vi "string_to_numberVariant.vi"(11 "String":string) -> (0 "error out":errorcluster, 3 "Variant":variant)   [LabVIEW 2014]
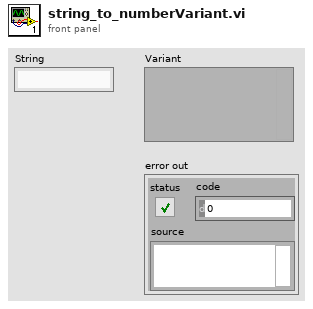
[diagram p1: front panel]
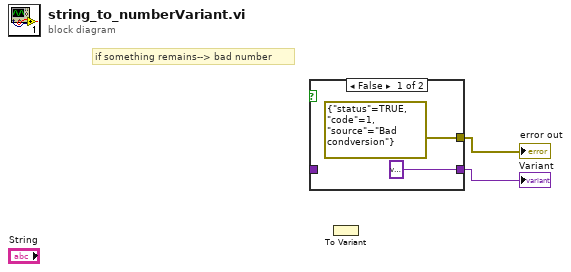
[diagram p0: block diagram]
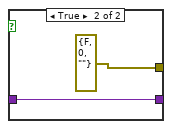
[diagram p2: hidden frame]
diagram:
  # "if something remains--> bad number"
  n1 = case shown="False" w2 {
    tunnel: [variant w10] -> w6
    tunnel: _ -> [_ w10]
    tunnel: [errorcluster {"status"=TRUE, "code"=1, "source"="Bad condversion"} ("error IO") errorcluster {"status"=FALSE, "code"=0, "source"=""} ("error IO")] -> w5
    frame False {
    }
    frame True {
    }
  }
  "Variant" <- w6
  "error out" <- w5
  n2 = To Variant() -> (anything=w1:cluster{}, Variant=w3:variant)
